vi "Acquire Host Key Database.vi"(8 "error in (no error)":errorcluster, 11 "host key database":T1) -> (0 "error out":errorcluster, 2 "LIBSSH2_KNOWNHOSTS*":u64)   [LabVIEW 2013, in "libssh2.lvlib"]
uses:
  libssh2.lvlib
  Host Key Database Refnum.ctl
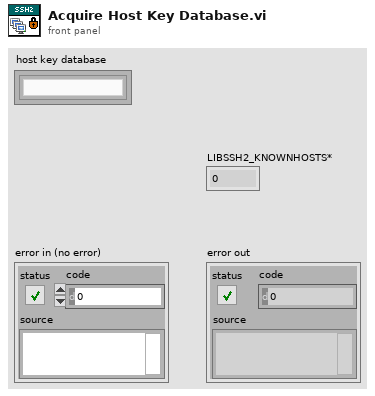
[diagram p1: front panel]
types:
  T1 = typedef "libssh2.lvlib/Host Key Database Refnum.ctl" = refnum<k1>
  T2 = typedef "Semaphore RefNum" = refnum<k1>
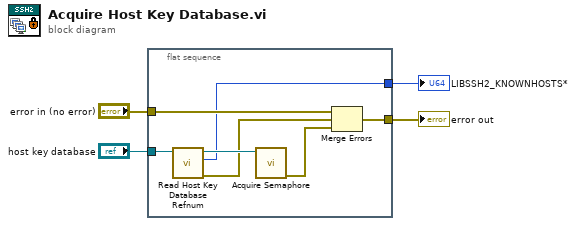
[diagram p0: block diagram]
diagram:
  n1 = flat-sequence {
    tunnel: [w8] -> w4
    tunnel: "error in (no error)" -> [w7]
    tunnel: "host key database" -> [w6]
    tunnel: [w5] -> w1
    frame #0 {
      n2 = call "Read Host Key Database Refnum.vi"("host key database"=w6) -> ("error out"=w10:errorcluster, "LIBSSH2_KNOWNHOSTS*"=w5:u64, "semaphore"=w11:T2)  [unwired: 8 in]
      n3 = call <vilib>:"Acquire Semaphore.vi"("semaphore"=w11) -> ("error out"=w9:errorcluster)  [unwired: 4 in, 2 out]
      n4 = Merge Errors(w7, w10, w9) -> (w8:errorcluster)
    }
  }
  "error out" <- w4
  "LIBSSH2_KNOWNHOSTS*" <- w1
